vi "specu1a 1.0.0 Open by Class or Name.vi"(3 "error in":errorcluster, 4 "Unit ID":string, 5 "specu1a 1.0.0 Model Class":T2) -> (0 "error out":errorcluster, 1 "Unit Information out":T1={"UnitID"="", "Sensor Name"="", "Serial Number"="", "Reserved"="", "Wave Upper"=630, "Wave Lower"=1050}, 2 "Device Handle":i32)   [LabVIEW 2010]
uses:
  Controls/specu1a 1.0.0 Model Class.ctl
  Controls/specu1a 1.0.0 Product Information.ctl
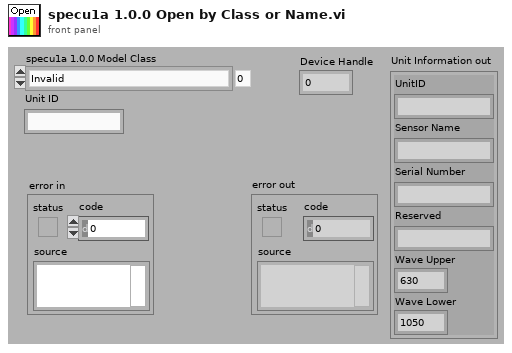
[diagram p1: front panel]
types:
  T1 = typedef "specu1a 1.0.0 Product Information.ctl" = cluster{"UnitID":string, "Sensor Name":string, "Serial Number":string, "Reserved":string, "Wave Upper":u16, "Wave Lower":u16}
  T2 = typedef "specu1a 1.0.0 Model Class.ctl" = enum16{"Invalid", "TG-NIR or SWNIR or UV", "TG-COOLED NIR-I or II", "TM-UV/VIS or VIS/NIR", "TM-UV/VIS or VIS/NIR CCD1 or CCD2", "RC- Vis or SWNIR Module"}
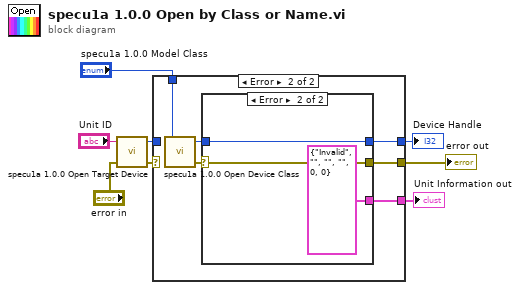
[diagram p0: block diagram]
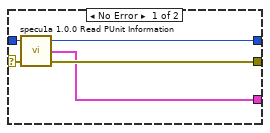
[diagram p2: hidden frame]
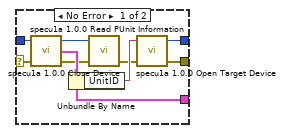
[diagram p3: hidden frame]
diagram:
  n1 = call "specu1a 1.0.0 Open Target Device.vi"("error in"="error in", "Unit ID"="Unit ID") -> ("error out"=w3:errorcluster, "Device Handle"=w2:i32)  [unwired: 1 in, 1 out]
  n2 = case shown="Error" w3 {
    selector: w3 -> [w12 _]
    tunnel: [w10 w17] -> w6
    tunnel: w2 -> [w13 _]
    tunnel: [w11 w16] -> w5
    tunnel: "specu1a 1.0.0 Model Class" -> [_ w14]
    tunnel: [w9 w15] -> w4
    frame No Error {
      n3 = call "specu1a 1.0.0 Read PUnit Information.vi"("error in (no error)"=w12, "Device Handle"=w13) -> ("error out"=w10:errorcluster, "Unit Information out"=w9:T1, "Device Handle out"=w11:i32)  [unwired: 1 in]
    }
    frame Error {
      n4 = call "specu1a 1.0.0 Open Device Class.vi"("specu1a 1.0.0 Model Name"=w14) -> ("error out"=w18:errorcluster, "Device Handle"=w19:i32)  [unwired: 3 in]
      n5 = case shown="Error" w18 {
        selector: w18 -> [w27 w31]
        tunnel: w19 -> [w28 w30]
        tunnel: [w22 w31] -> w17
        tunnel: [w23 w30] -> w16
        tunnel: [w26 T1 {"UnitID"="Invalid", "Sensor Name"="", "Serial Number"="", "Reserved"="", "Wave Upper"=0, "Wave Lower"=0} ("Unit Information out")] -> w15
        frame No Error {
          n6 = call "specu1a 1.0.0 Read PUnit Information.vi"("error in (no error)"=w27, "Device Handle"=w28) -> ("error out"=w21:errorcluster, "Unit Information out"=w26:T1, "Device Handle out"=w25:i32)  [unwired: 1 in]
          n7 = Unbundle By Name(w26) -> ("UnitID"=w24:string)
          n8 = call "specu1a 1.0.0 Close Device.vi"("error in (no error)"=w21, "Device Handle"=w25) -> ("error out"=w20:errorcluster)  [unwired: 3 in]
          n9 = call "specu1a 1.0.0 Open Target Device.vi"("error in"=w20, "Unit ID"=w24) -> ("error out"=w22:errorcluster, "Device Handle"=w23:i32)  [unwired: 1 in, 1 out]
        }
        frame Error {
        }
      }
    }
  }
  "error out" <- w6
  "Device Handle" <- w5
  "Unit Information out" <- w4
